vi "Free Running Avs47b.vi"() -> ()   [LabVIEW 2012]
doc: "Application example"
panel:
  in  "stop":bool
  out "RESISTANCE":sgl format="%^_6e"
  in  "REMOTE":u8(ring)=1 items=["NO", "YES"]
  in  "DIGITAL REFERENCE":u16 max=19999 step=1
  in  "DISPLAY":u8(ring) items=["R", "DR", "ADJ REF", "REFERENCE", "EXC VOLT", "530A HEAT V", "530A HEAT I", "530A SET PT"]
  in  "EXCITATION":u8(ring)=7 items=["NO EXCITATION", "3 uV", "10uV", "30uV", "100uV", "300uV", "1mV", "3mV"]
  in  "RANGE":u8(ring)=3 items=["NO RANGE", "2 Ohms", "20 Ohms", "200 Ohms", "2 kOhms", "20 kOhms", "200 kOhms", "2 MOhms"]
  in  "CHANNEL":u8(ring) items=["CH0", "CH1", "CH2", "CH3", "CH4", "CH5", "CH6", "CH7"]
  in  "INPUT":u8(ring)=2 items=["ZERO", "MEAS", "CAL"]
  out "ADC OVERRANGE":bool
  # "FreeRunningAvs47b.vi"
  # "Ohms"
  # "This rather simple applicaton example shows, how a continuously running VI can be used\nfor producing readings to be read by another VIs when needed.\n\nSettings are read from the configuration file.  Storing them to local variables makes them\nwork as initial values for the controls.  The the program enters into a while loop, where\nyou can change the settings. The AVS-47B is configured (if in remote) and the A/D converter is \nread.  Resistance readings are stored in a functional grobal variable (VI) 2.5 times/s, when its \ncontrol input is \"set resistance\".  You can read the last stored resistance value by running a \nsecond copy of this global somewhere in your application when the control input is set to \n\"read resistance\".\n\nThis VI starts always in the local mode for safety."
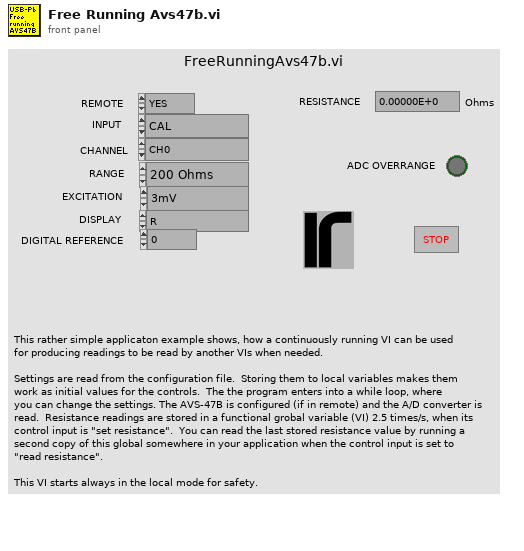
[diagram p1: front panel]
types:
  T1 = cluster{"VISA RESOURCE":refnum<visa-resource-name>, "PICOBUS ADDRESS":u8, "DISABLE AL":u8, "REMOTE":u8, "INPUT":u8, "CHANNEL":u8, "RANGE":u8, "EXCITATION":u8, "DISPLAY":u8, "DIGITAL REFERENCE":u16, "SET POINT":dbl, "PROP GAIN":u8, "INTG":u8, "DERIV":u8, "POWER BIAS":u8, "POWER RANGE":u8, "INFO STRING":string, "HEATER RESISTANCE":dbl, "INTERVAL":u8, " SENSOR dR/dT":u8}
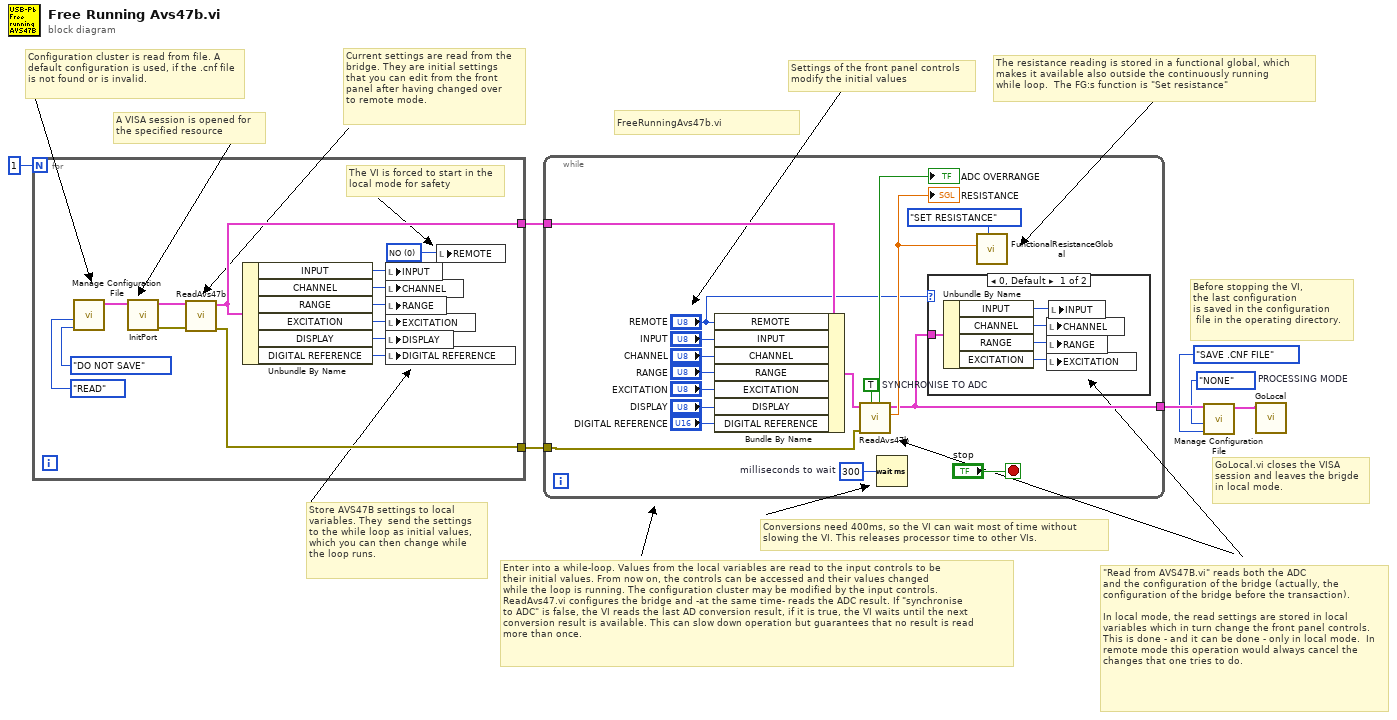
[diagram p0: block diagram]
diagram:
  w2 = enum16{"NONE", "READ", "CREATE"}."NONE"  # PROCESSING MODE
  # "A VISA session is opened for\nthe specified resource"
  # "Current settings are read from the\nbridge. They are initial settings\nthat you can edit from the front\npanel after having changed over\nto remote mode."
  # "\"Read from AVS47B.vi\" reads both the ADC\nand the configuration of the bridge (actually, the configuration of the bridge before the transaction).\n\nIn local mode, the read settings are stored in local variables which in turn change the front panel controls. This is done - and it can be done - only in local mode.  In remote mode this operation would always cancel the changes that one tries to do."
  # "Conversions need 400ms, so the VI can wait most of time without\nslowing the VI. This releases processor time to other VIs."
  # "Settings of the front panel controls\nmodify the initial values"
  # "Configuration cluster is read from file. A default configuration is used, if the .cnf file is not found or is invalid."
  # "GoLocal.vi closes the VISA\nsession and leaves the brigde\nin local mode."
  # "Before stopping the VI,\nthe last configuration\nis saved in the configuration\n file in the operating directory."
  # "The resistance reading is stored in a functional global, which\nmakes it available also outside the continuously running \nwhile loop.  The FG:s function is \"Set resistance\""
  # "Enter into a while-loop. Values from the local variables are read to the input controls to be\ntheir initial values. From now on, the controls can be accessed and their values changed\nwhile the loop is running. The configuration cluster may be modified by the input controls.\nReadAvs47.vi configures the bridge and -at the same time- reads the ADC result. If \"synchronise\nto ADC\" is false, the VI reads the last AD conversion result, if it is true, the VI waits until the next\nconversion result is available. This can slow down operation but guarantees that no result is read \nmore than once."
  # "Store AVS47B settings to local\nvariables. They  send the settings\nto the while loop as initial values,\nwhich you can then change while\nthe loop runs."
  # "FreeRunningAvs47b.vi"
  n1 = for {
    N: 1 -> [_]
    tunnel: [w12] -> w6
    tunnel: [w14] -> w5
    w15 = u8 0 items=["NO", "YES"] ("REMOTE")
    # "The VI is forced to start in the\nlocal mode for safety"
    n2 = call "Manage Configuration File.vi"("SAVE MODE"=enum16{"DO NOT SAVE", "SAVE .CNF FILE"}."DO NOT SAVE", "PROCESSING MODE"=enum16{"NONE", "READ", "CREATE"}."READ") -> ("CONFIGURATION CLUSTER OUT"=w11:T1)  [unwired: 9 in]
    n3 = call "InitPort.vi"("CONFIGURATION CLUSTER"=w11) -> ("LV ERROR OUT"=w13:errorcluster, "UNMODIFIED CONFIGURATION CLUSTER"=w10:T1)  [unwired: 6 in, 1 out]
    n4 = call "ReadAvs47b.vi"("LV ERROR IN"=w13, "CONFIGURATION CLUSTER"=w10) -> ("LV ERROR OUT"=w12:errorcluster, "MODIFIED CONFIGURATION CLUSTER"=w14:T1)  [unwired: 4 in, 4 out]
    n5 = Unbundle By Name(w14) -> ("INPUT"=w21:u8, "CHANNEL"=w20:u8, "RANGE"=w19:u8, "EXCITATION"=w18:u8, "DISPLAY"=w17:u8, "DIGITAL REFERENCE"=w16:u16)
    n6 = local write "INPUT"(w21) -> ()
    n7 = local write "CHANNEL"(w20) -> ()
    n8 = local write "RANGE"(w19) -> ()
    n9 = local write "EXCITATION"(w18) -> ()
    n10 = local write "DISPLAY"(w17) -> ()
    n11 = local write "DIGITAL REFERENCE"(w16) -> ()
    n12 = local write "REMOTE"(w15) -> ()
  }
  n13 = while {
    tunnel: w6 -> [w38]
    tunnel: [w24] -> w3
    tunnel: w5 -> [w28]
    stop <- "stop" stop-if-true
    w22 = TRUE  # SYNCHRONISE TO ADC
    w37 = u32 300  # milliseconds to wait
    n14 = Bundle By Name(cluster=w28, "REMOTE"="REMOTE", "INPUT"="INPUT", "CHANNEL"="CHANNEL", "RANGE"="RANGE", "EXCITATION"="EXCITATION", "DISPLAY"="DISPLAY", "DIGITAL REFERENCE"="DIGITAL REFERENCE") -> (w36:T1)
    n15 = call "ReadAvs47b.vi"("SYNCHRONISE TO ADC"=w22, "LV ERROR IN"=w38, "CONFIGURATION CLUSTER"=w36) -> ("RESISTANCE (OHMS)"=w26:sgl, "MODIFIED CONFIGURATION CLUSTER"=w24:T1, "ADC OVERRANGE"=→"ADC OVERRANGE":bool)  [unwired: 3 in, 3 out]
    "RESISTANCE" <- w26
    n16 = Wait (ms)(milliseconds to wait=w37) -> ()  [unwired: 1 out]
    n17 = case shown="0, Default" "REMOTE" {
      tunnel: w24 -> [w43 _]
      frame 0, Default {
        n18 = Unbundle By Name(w43) -> ("INPUT"=w42:u8, "CHANNEL"=w41:u8, "RANGE"=w40:u8, "EXCITATION"=w39:u8)
        n19 = local write "CHANNEL"(w41) -> ()
        n20 = local write "RANGE"(w40) -> ()
        n21 = local write "EXCITATION"(w39) -> ()
        n22 = local write "INPUT"(w42) -> ()
      }
      frame 1 {
      }
    }
    n23 = call "FunctionalResistanceGlobal.vi"("FUNCTION"=enum16{"SET RESISTANCE", "READ RESISTANCE"}."SET RESISTANCE", "RESISTANCE IN"=w26) -> ()  [unwired: 9 in, 1 out]
  }
  n24 = call "Manage Configuration File.vi"("SAVE MODE"=enum16{"DO NOT SAVE", "SAVE .CNF FILE"}."SAVE .CNF FILE", "PROCESSING MODE"=w2, "CONFIGURATION CLUSTER"=w3) -> ("CONFIGURATION CLUSTER OUT"=w4:T1)  [unwired: 8 in]
  n25 = call "GoLocal.vi"("CONFIGURATION CLUSTER"=w4) -> ()  [unwired: 10 in, 1 out]
